vi "Draw_Shape_Circles.vi"(6 "Color":u32(colorbox)=16711680, 8 "error in":errorcluster, 10 "Circle Descriptor":T1, 11 "Image":T2) -> (0 "error out":errorcluster, 3 "Image Out":T2)   [LabVIEW 2019]
uses:
  <vilib>/vision/Image Controls.llb/IMAQ Image.ctl
panel:
  in  "Group":string
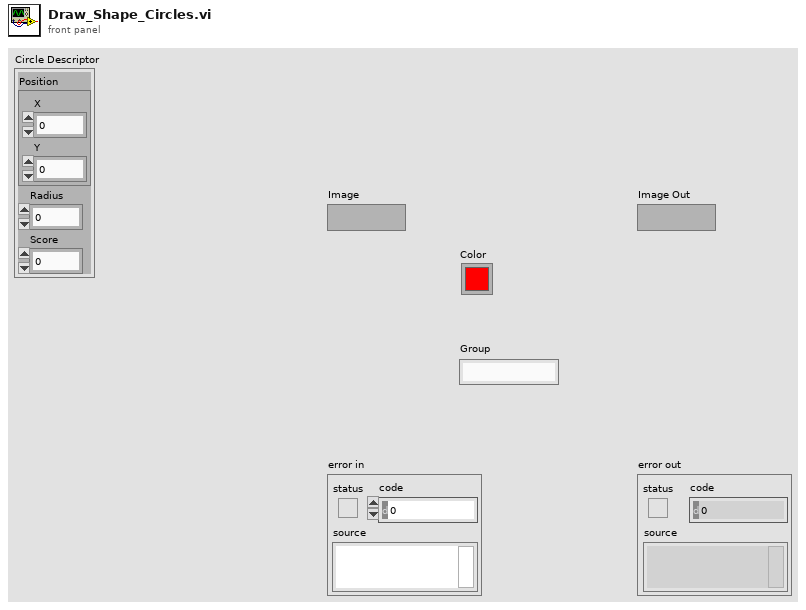
[diagram p1: front panel]
types:
  T1 = cluster{"Position":cluster{"X":sgl, "Y":sgl}, "Radius":dbl, "Score":dbl}
  T2 = typedef "IMAQ Image.ctl" = refnum<image>
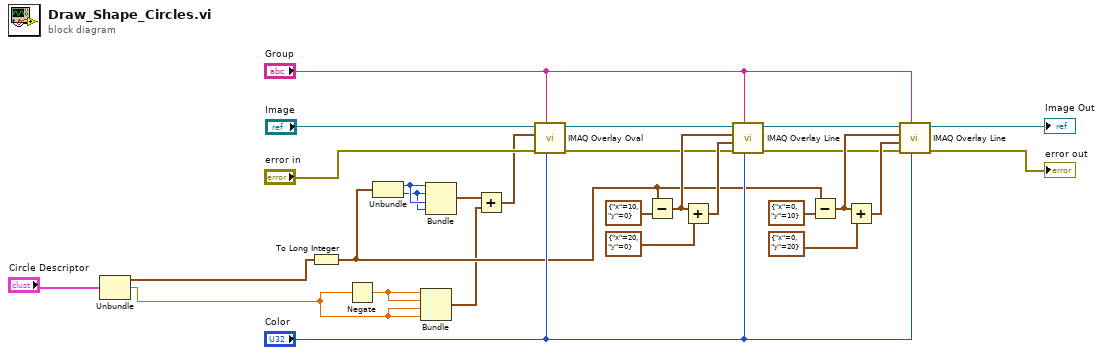
[diagram p0: block diagram]
diagram:
  n1 = Unbundle("Circle Descriptor") -> ("Position"=w3:cluster{"X":sgl, "Y":sgl}, "Radius"=w2:dbl)  [unwired: 1 out]
  n2 = To Long Integer(number=w3) -> (32bit integer=w8:cluster{"X":i32, "Y":i32})
  n3 = Negate(x=w2) -> (-x=w1:dbl)
  n4 = Unbundle(w8) -> ("X"=w23:i32, "Y"=w22:i32)
  n5 = Bundle(w1, w1, "Radius"=w2, "Radius"=w2) -> (w5:cluster{dbl, dbl, "Radius":dbl, "Radius":dbl})  [unwired: 1 in]
  n6 = Bundle("X"=w23, "Y"=w22, "X"=w23, "Y"=w22) -> (w21:cluster{"X":i32, "Y":i32, "X":i32, "Y":i32})  [unwired: 1 out]
  n7 = Add(x=w21, y=w5) -> (x+y=w20:cluster{dbl, dbl, dbl, dbl})
  n8 = call "IMAQ Overlay Oval"("Color"="Color", "Group"="Group", "error in (no error)"="error in", "Bounding Rectangle"=w20, "Image"="Image") -> ("error out"=w10:errorcluster, "Image Out"=w24:T2)  [unwired: 1 in, 4 out]
  n9 = Subtract(x=w8, y=cluster{"x":i32, "y":i32} {"x"=10, "y"=0}) -> (x-y=w18:cluster{i32, i32})
  n10 = Add(x=w18, y=cluster{"x":i32, "y":i32} {"x"=20, "y"=0}) -> (x+y=w16:cluster{i32, i32})
  n11 = call "IMAQ Overlay Line"("Color"="Color", "Group"="Group", "error in (no error)"=w10, "End Point"=w16, "Start Point"=w18, "Image"=w24) -> ("error out"=w9:errorcluster, "Image Out"=w11:T2)  [unwired: 4 out]
  n12 = Subtract(x=w8, y=cluster{"x":i32, "y":i32} {"x"=0, "y"=10}) -> (x-y=w14:cluster{i32, i32})
  n13 = Add(x=w14, y=cluster{"x":i32, "y":i32} {"x"=0, "y"=20}) -> (x+y=w15:cluster{i32, i32})
  n14 = call "IMAQ Overlay Line"("Color"="Color", "Group"="Group", "error in (no error)"=w9, "End Point"=w15, "Start Point"=w14, "Image"=w11) -> ("error out"=→"error out":errorcluster, "Image Out"=→"Image Out":T2)  [unwired: 4 out]
